vi "GP22_TDC_Arduinoed Measurement.vi"() -> ()   [LabVIEW 2013, in "GP22_TDC_Arduinoed.lvlib"]
uses:
  GP22_TDC_Arduinoed.lvlib
  <vilib>/Utility/file.llb/Write To Spreadsheet File (DBL).vi
  Public/Globals.vi
  <vilib>/Analysis/NI_AALBase.lvlib
panel:
  out "Calibration":dbl[](array[numeric])
  out "Raw output":dbl[](array[numeric])
  in  "Time between calibrations (ms)":u32=1000
  out "Mean Time / s":dbl format="%^.3e"
  out "Histogram":dynamicdata(graph)
  out "Time frac. S.D.":dbl
  out "Mean Freq / Hz":dbl
  out "Size":i32
  out "output/s":dbl[](array[numeric]) format="%^#_6g"
  in  "Time in ms (30000)":u32=30000
  out "error out":errorcluster
  out "Self-Test Result Message":string
  in  "VISA resource name":refnum<visa-resource-name>="COM6"
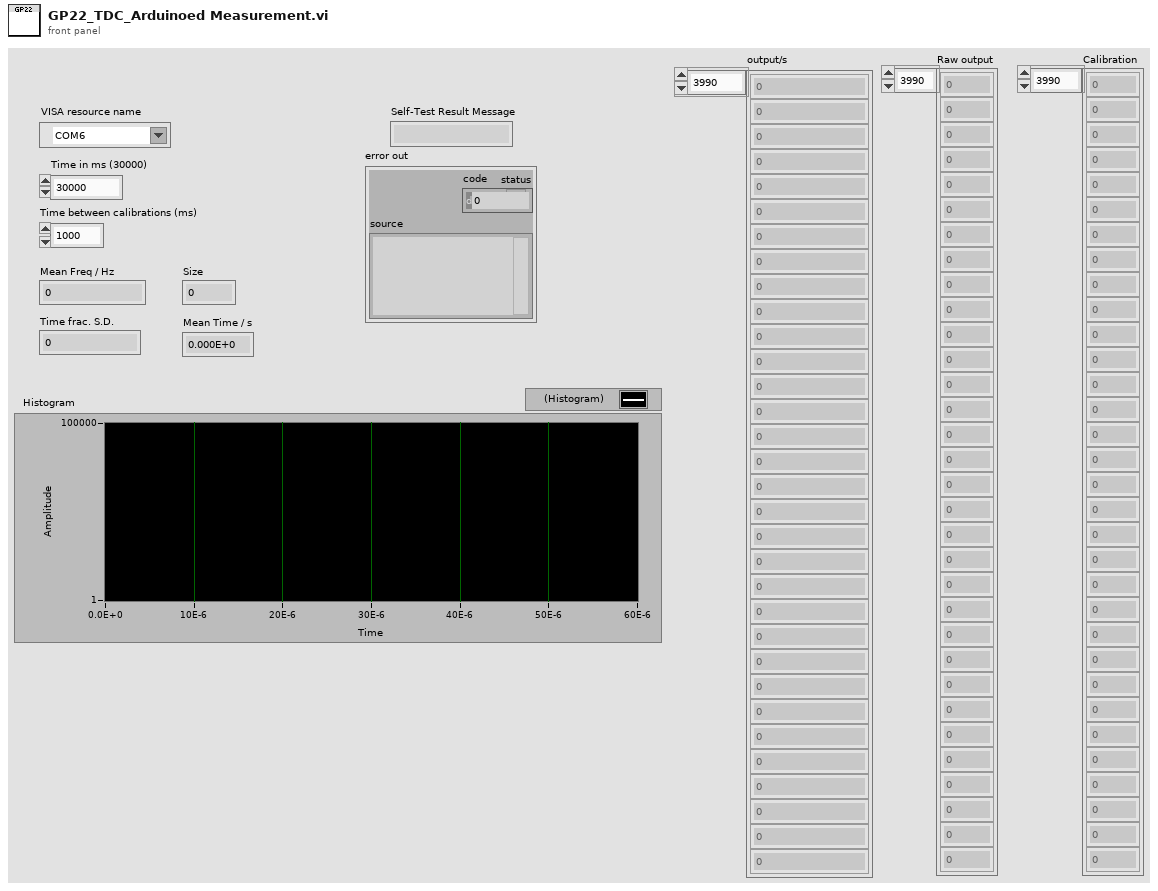
[diagram p1: front panel]
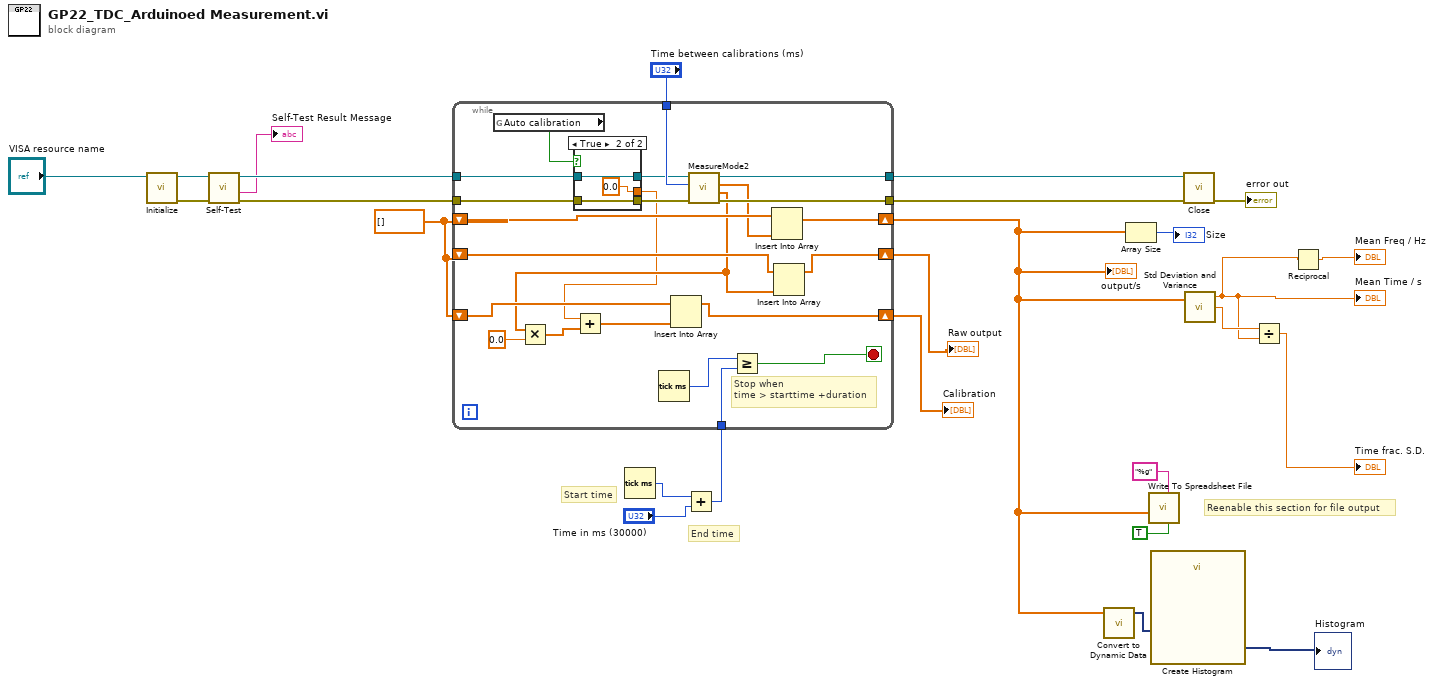
[diagram p0: block diagram]
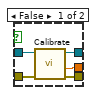
[diagram p2: hidden frame]
diagram:
  w2 = dbl[] [] ("output")
  # "End time"
  # "Start time"
  # "Reenable this section for file output"
  n1 = call "Initialize.vi"("VISA resource name"="VISA resource name") -> ("error out"=w23:errorcluster, "VISA resource name out"=w25:refnum<visa-resource-name>)  [unwired: 9 in]
  n2 = call "Self-Test.vi"("error in (no error)"=w23, "VISA resource name"=w25) -> ("error out"=w11:errorcluster, "Self-Test Result Message"=→"Self-Test Result Message":string, "VISA resource name out"=w24:refnum<visa-resource-name>)  [unwired: 6 in, 1 out]
  n3 = Tick Count (ms)() -> (millisecond timer value=w9:u32)
  n4 = Add(x=w9, y="Time in ms (30000)") -> (x+y=w7:u32)
  n5 = while {
    tunnel: w24 -> [w43]
    tunnel: [w49] -> w20
    tunnel: "Time between calibrations (ms)" -> [w48]
    tunnel: w11 -> [w42]
    tunnel: [w47] -> w10
    tunnel: w7 -> [w45]
    shift-right: [w37] -> w17
    shift-left: w2 -> [w39]
    shift-right: [w34] -> w5
    shift-left: w2 -> [w35]
    shift-right: [w32] -> w1
    shift-left: w2 -> [w33]
    stop <- w44 stop-if-true
    # "Stop when \ntime > starttime +duration"
    n6 = global read "Globals.vi" "Auto calibration"() -> (w36:bool)
    n7 = case shown="True" w36 {
      tunnel: w43 -> [w54 w57]
      tunnel: w42 -> [w53 w56]
      tunnel: [w52 w56] -> w41
      tunnel: [w51 w57] -> w40
      tunnel: [w50 0.0 ("y")] -> w28
      frame False {
        n8 = call "Calibrate.vi"("error in (no error)"=w53, "VISA resource name"=w54) -> ("error out"=w52:errorcluster, "output raw"=w50:dbl, "VISA resource name out"=w51:refnum<visa-resource-name>)  [unwired: 5 in, 1 out]
      }
      frame True {
      }
    }
    n9 = Tick Count (ms)() -> (millisecond timer value=w46:u32)
    n10 = call "MeasureMode2.vi"("error in (no error)"=w41, "Time in ms (30000)"=w48, "VISA resource name"=w40) -> ("error out"=w47:errorcluster, "Raw output"=w31:dbl[], "output/s"=w38:dbl[], "VISA resource name out"=w49:refnum<visa-resource-name>)  [unwired: 5 in]
    n11 = Multiply(x=w31, y=0.0) -> (x*y=w29:dbl[])
    n12 = Add(x=w28, y=w29) -> (x+y=w27:dbl[])
    n13 = Insert Into Array(array=w33, new element=w27) -> (w32:dbl[])  [unwired: 1 in]
    n14 = Greater Or Equal?(x=w46, y=w45) -> (x >= y?=w44:bool)
    n15 = Insert Into Array(array=w39, new element=w38) -> (w37:dbl[])  [unwired: 1 in]
    n16 = Insert Into Array(array=w35, new element=w31) -> (w34:dbl[])  [unwired: 1 in]
  }
  "output/s" <- w17
  "Raw output" <- w5
  "Calibration" <- w1
  n17 = call "Convert to Dynamic Data"("Array"=w17) -> ("Dynamic Data Type"=w16:dynamicdata)  [unwired: 3 in]
  n18 = Array Size(array=w17) -> (size(s)=→"Size":i32)
  n19 = call-poly <vilib>:"Write To Spreadsheet File.vi"("transpose? (no:F)"=TRUE, "format (%.3f)"="%g", "1D data"=w17) -> ()  [unwired: 5 in, 1 out]
  n20 = call "Create Histogram"("Signal"=w16) -> ("Histogram"=→"Histogram":dynamicdata)  [unwired: 9 in, 1 out]
  n21 = call "Close.vi"("error in (no error)"=w10, "VISA resource name"=w20) -> ("error out"=→"error out":errorcluster)  [unwired: 9 in]
  n22 = call <vilib>:"Std Deviation and Variance.vi"("X"=w17) -> ("mean"=w12:dbl, "standard deviation"=w14:dbl)  [unwired: 1 in, 1 out]
  "Mean Time / s" <- w12
  n23 = Divide(x=w14, y=w12) -> (x/y=→"Time frac. S.D.":dbl)
  n24 = Reciprocal(x=w12) -> (1/x=→"Mean Freq / Hz":dbl)
